vi "smooth curve.vi"(2 "balance parameter":dbl=-1.0, 3 "discrete points":cluster{"x":dbl, "y":dbl}[](array[cluster]), 4 "data points":i32=100) -> (0 "y":dbl[](array[numeric]), 1 "x":dbl[](array[numeric]))   [LabVIEW 2009]
uses:
  <vilib>/Analysis/NI_AALPro.lvlib
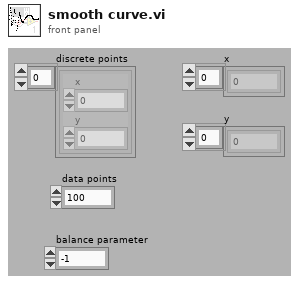
[diagram p1: front panel]
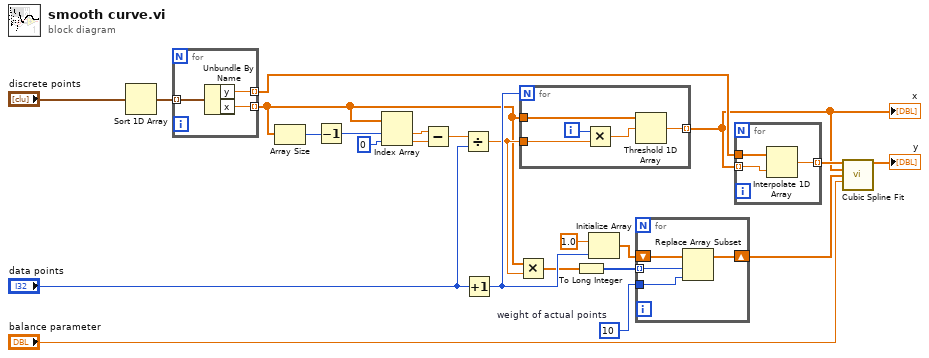
[diagram p0: block diagram]
diagram:
  w7 = 10  # weight of actual points
  n1 = Sort 1D Array(array="discrete points") -> (sorted array=w1:cluster{"x":dbl, "y":dbl}[])
  n2 = for {
    tunnel: w1 -> [w26] mode=indexing
    tunnel: [w25] -> w11 mode=indexing
    tunnel: [w24] -> w12 mode=indexing
    n3 = Unbundle By Name(w26) -> ("y"=w25:dbl, "x"=w24:dbl)
  }
  n4 = Array Size(array=w12) -> (size(s)=w21:i32)
  n5 = Decrement(x=w21) -> (x-1=w20:i32)
  n6 = Index Array(array=w12, index #1=w20, index #2=0 ("index")) -> (element #1=w19:dbl, element #2=w18:dbl)
  n7 = Subtract(x=w19, y=w18) -> (x-y=w17:dbl)
  n8 = Divide(x=w17, y="data points") -> (x/y=w13:dbl)
  n9 = Increment(x="data points") -> (x+1=w15:i32)
  n10 = Multiply(x=w12, y=w13) -> (x*y=w10:dbl[])
  n11 = for {
    N: w15 -> [_]
    tunnel: w12 -> [w31]
    tunnel: [w30] -> w2 mode=indexing
    tunnel: w13 -> [w28]
    i -> [w29]
    n12 = Multiply(x=w29, y=w28) -> (x*y=w27:dbl)
    n13 = Threshold 1D Array(2:w27, 3:w31) -> (0:w30:dbl)  [unwired: 1 in]
  }
  "x" <- w2
  n14 = To Long Integer(number=w10) -> (32bit integer=w8:i32[])
  n15 = Initialize Array(1.0 ("element"), w15) -> (w9:dbl[])
  n16 = for {
    shift-right: [w34] -> w5
    shift-left: w9 -> [w35]
    tunnel: w8 -> [w33] mode=indexing
    tunnel: w7 -> [w32]
    n17 = Replace Array Subset(array=w35, new element=w32, index=w33) -> (w34:dbl[])
  }
  n18 = for {
    tunnel: w2 -> [w38] mode=indexing
    tunnel: w11 -> [w37]
    tunnel: [w36] -> w6 mode=indexing
    n19 = Interpolate 1D Array(1:w38, 2:w37) -> (0:w36:dbl)
  }
  n20 = call <vilib>:"Cubic Spline Fit.vi"("Y"=w6, "X"=w2, "Weight"=w5, "balance parameter"="balance parameter") -> ("Best Cubic Spline Fit"=→"y":dbl[])  [unwired: 10 in, 1 out]
